vi "Set Render Prio.vi"(8 "error in (no error)":errorcluster, 10 "Low Prio Rendering":T1, 11 "Signal Analysis in":refnum<class "Signal Analysis.lvclass">) -> (0 "error out":errorcluster, 3 "Signal Analysis out":refnum<class "Signal Analysis.lvclass">)   [LabVIEW 2020, in "Signal Analysis.lvlib" / "Signal Analysis.lvclass"]
uses:
  Signal Analysis.lvclass
  Low Prio Rendering.ctl
  Helper Loop Message.ctl
  Helper Loop Type.ctl
  Signal Analysis.lvclass/Signal Analysis.ctl
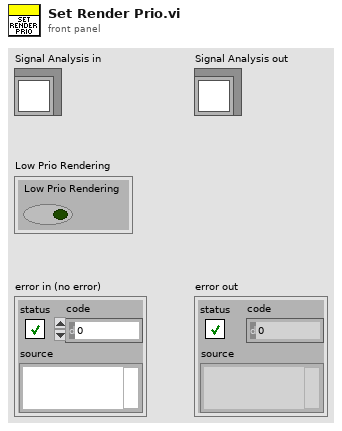
[diagram p1: front panel]
types:
  T1 = typedef "Signal Analysis.lvlib/Signal Analysis.lvclass/Low Prio Rendering.ctl" = cluster{"Low Prio Rendering":bool}
  T2 = typedef "Signal Analysis.lvlib/Signal Analysis.lvclass/Helper Loop Message.ctl" = cluster{"Type":T3, "Payload":variant}
  T3 = typedef "Signal Analysis.lvlib/Signal Analysis.lvclass/Helper Loop Type.ctl" = enum16{"Process Data", "Set Batch Size", "Set Render Prio", "Close", "Set FFT Size"}
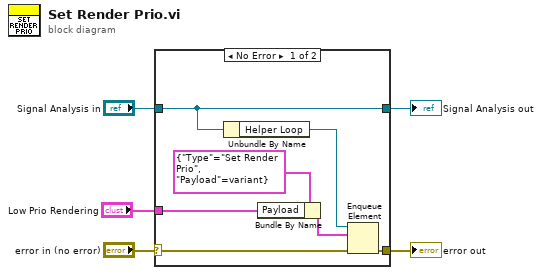
[diagram p0: block diagram]
diagram:
  n1 = case shown="No Error" "error in (no error)" {
    selector: "error in (no error)" -> [w11 w14]
    tunnel: [w12 w14] -> w4
    tunnel: [w10 w13] -> w2
    tunnel: "Signal Analysis in" -> [w10 w13]
    tunnel: "Low Prio Rendering" -> [w6 _]
    frame No Error {
      n2 = Unbundle By Name(w10) -> ("Helper Loop"=w9:refnum<queue>)
      n3 = Bundle By Name(cluster=T2 {"Type"=enum."Set Render Prio", "Payload"=variant} ("element"), "Payload"=w6) -> (w7:T2)
      n4 = Enqueue Element(queue=w9, element=w7, error in (no error)=w11) -> (error out=w12:errorcluster)  [unwired: 1 in, 2 out]
    }
    frame Error {
    }
  }
  "error out" <- w4
  "Signal Analysis out" <- w2
